vi "Acquire Every Image (178x Smart Camera).vi"() -> ()   [LabVIEW 2023]
doc: "The Acquire Every Image (178x Smart Camera) example performs a high-level grab acquisition and exposes control of the sensor interface for ISC-178x smart cameras. A grab is appropriate for high-speed applications that process only one image at a time.\n\nUse the <B>Sensor Parameters</B> cluster to control attributes related to the sensor. Use the <B>Exposure Time (ms)</B> control to precisely control the amount of time (in milliseconds) that the image sensor is sensitive to light. Use the <B>Gain</B> control to determine the gain of the camera. Use the <B>Reverse X</B> and <B>Reverse Y</B> to flip the image horizontally or vertically.\n\nUse the <B>Lighting Parameters</B> cluster to control the strobe and lighting intensity raw analog output value. The strobe output signal can be output on any ISO output line and is precisely synchronized with the exposure of the image sensor. This guarantees that the light is on for the duration of the image exposure period. The <B>Lighting Intensity Raw</B> is an analog output that can adjust the intensity of a light. \n\nUse the <B>Trigger Parameters</B> cluster to configure the trigger mode of the acquisition. These settings must be configured before running the VI because they are ignored while the acquisition is active."
uses:
  <vilib>/vision/driver/IMAQdx.llb/IMAQdx Buffer Number Mode.ctl
  <vilib>/vision/driver/NI_Vision_Acquisition_Software.lvlib
  <resource>/objmgr/imaqdx.rc
panel:
  in  "SW Trigger":bool
  in  "Trigger Parameters":T1={"Trigger Mode"="Off", "Trigger Source"="Input 0", "Trigger Activation"="Rising Edge", "Acquisition Frame Rate"=1.0, "Timeout (ms)"=5000, "Trigger Delay (us)"=0.0} {"Trigger Delay (us)" min=0.0 max=0.0; "Acquisition Frame Rate" min=0.25 max=293.0}
  in  "Lighting Parameters":T2={"Strobe ISO Output Line"="Off", "Lighting Intensity Raw"=0} {"Lighting Intensity Raw" max=255 step=1 scale=0.0..255.0}
  in  "Color Parameters":T3 {"Blue Gain" scale=0.0..3.99; "Green Gain" scale=0.0..3.99; "Red Gain" scale=0.0..3.99}
  in  "Sensor Parameters":T4={"Exposure Time (ms)"=8.128, "Gain"=0.0, "Reverse X"=FALSE, "Reverse Y"=FALSE} {"Gain" min=0.0 max=255.0; "Exposure Time (ms)" min=0.0 max=4200.0 scale=0.05..4200.0 scale format="%#_1f"}
  in  "Camera Name":refnum<k21> caption="IMAQdx Session"
  out "Image":T5(plugin-control)
  out "Frame Rate":dbl=61.507936507936506 max=294.0
  in  "Stop":bool
  # "Overview: Demonstrates how to perform a high-level grab acquisition and control of the sensor interface for ISC-178x smart camera.  \nRequirements: Vision Acquisition Software, ISC-178x smart camera.\nInstructions: \n1. Open a new LabVIEW Project by selecting Project»Create Project. Select Add this VI when prompted to add this VI to the project.\n2. Right click on the top-level project item in the tree and select New»Targets and Devices\n3. Select the ISC-178x smart camera you want to run this example with, and click OK.\n4. Drag this VI from My Computer to the smart camera target.\n5. Double click on the example under the smart camera, select the Camera Name, and run the VI."
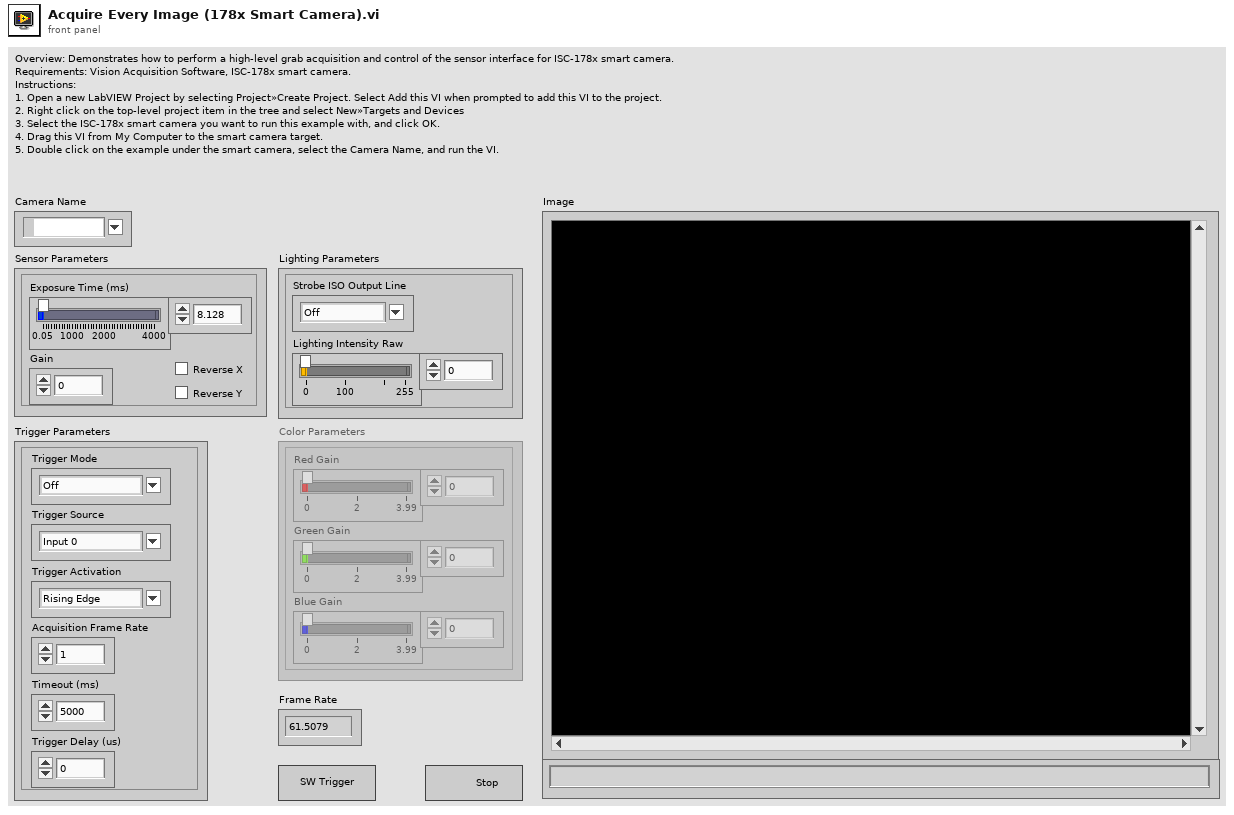
[diagram p1: front panel]
types:
  T1 = cluster{"Trigger Mode":string, "Trigger Source":string, "Trigger Activation":string, "Acquisition Frame Rate":dbl, "Timeout (ms)":u32, "Trigger Delay (us)":dbl}
  T2 = cluster{"Strobe ISO Output Line":string, "Lighting Intensity Raw":u32}
  T3 = cluster{"Red Gain":dbl, "Green Gain":dbl, "Blue Gain":dbl}
  T4 = cluster{"Exposure Time (ms)":dbl, "Gain":dbl, "Reverse X":bool, "Reverse Y":bool}
  T5 = typedef "IMAQ Image.ctl" = refnum<image>
  T6 = enum8{"Enabled", "Disabled", "Disabled and Grayed Out"}
  T7 = typedef "IMAQdx.ctl" = refnum<k21>
  T8 = typedef "NI_Vision_Acquisition_Software.lvlib/IMAQdx Buffer Number Mode.ctl" = enum32{"Next", "Last", "Buffer Number", "Every", "Last New"}
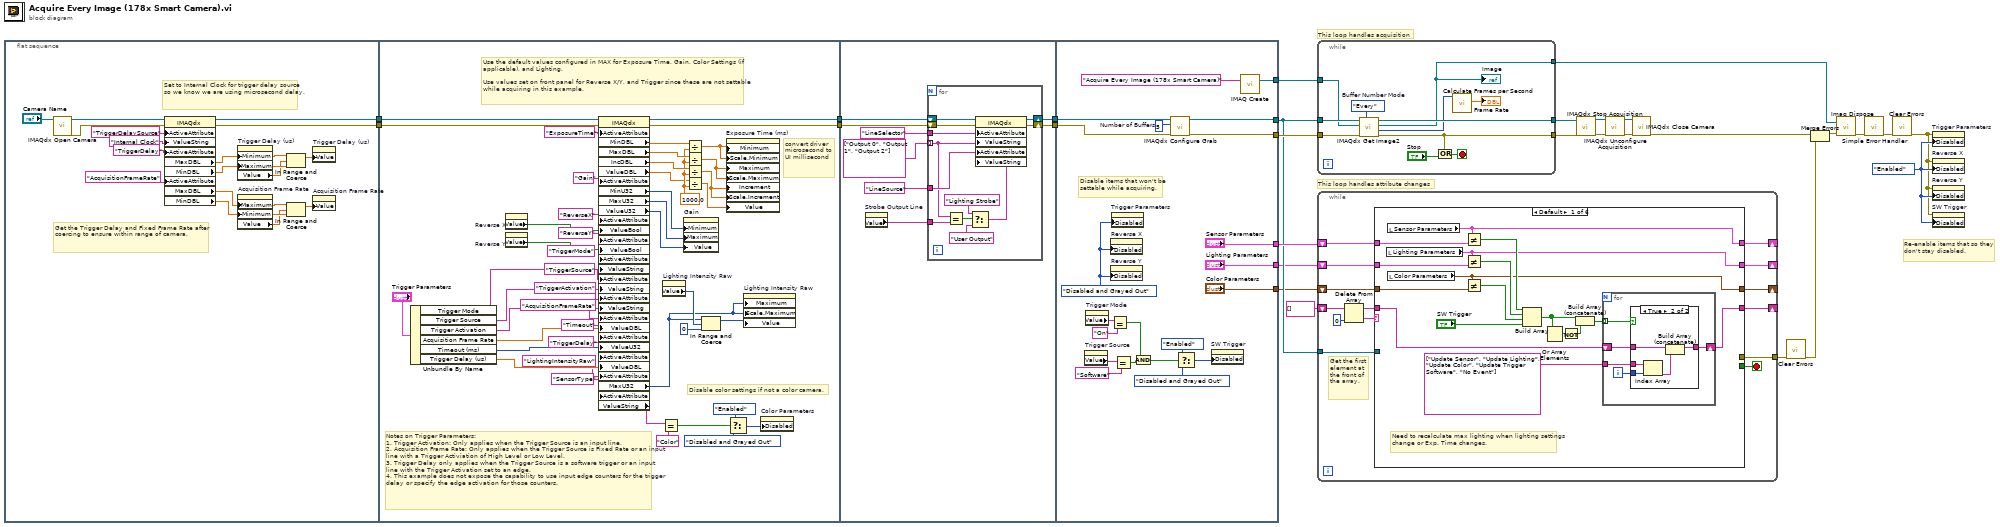
[diagram p0: block diagram]
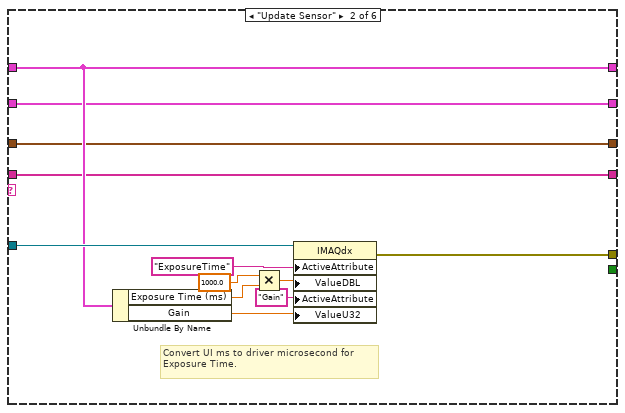
[diagram p3: hidden frame]
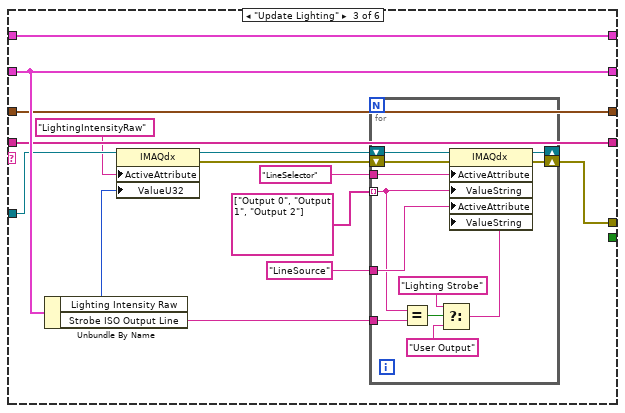
[diagram p4: hidden frame]
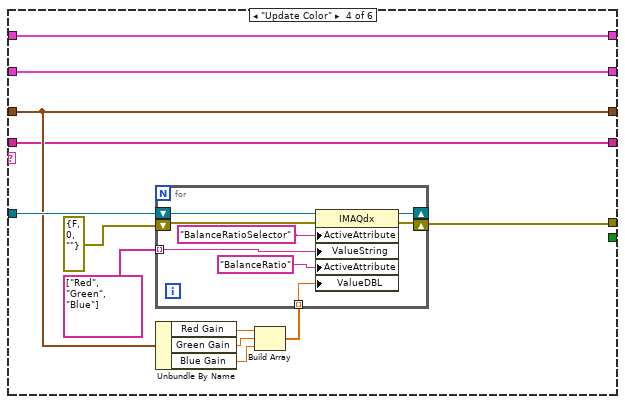
[diagram p5: hidden frame]
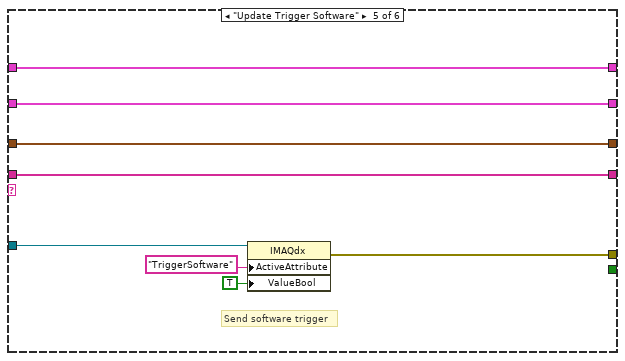
[diagram p6: hidden frame]
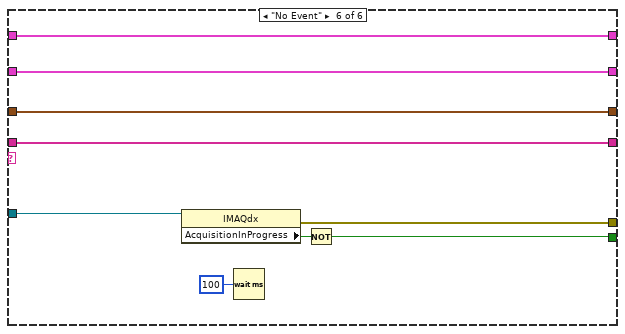
[diagram p7: hidden frame]
diagram:
  w16 = T6."Enabled" ("Disabled")
  # "Re-enable items that so they don't stay disabled."
  # "This loop handles acquisition"
  # "This loop handles attribute changes"
  n1 = flat-sequence {
    tunnel: [w32] -> w23
    tunnel: [w34] -> w22
    tunnel: w23 -> [w63]
    tunnel: [w62] -> w4
    tunnel: w22 -> [w82]
    tunnel: [w76] -> w2
    tunnel: w4 -> [w100]
    tunnel: [w98] -> w3
    tunnel: w2 -> [w99]
    tunnel: [w97] -> w1
    tunnel: w3 -> [w117]
    tunnel: [w116] -> w26
    tunnel: [w115] -> w28
    tunnel: ["Sensor Parameters"] -> w27
    tunnel: ["Lighting Parameters"] -> w25
    tunnel: ["Color Parameters"] -> w24
    tunnel: w1 -> [w114]
    tunnel: [w119] -> w21
    frame #0 {
      # "Get the Trigger Delay and Fixed Frame Rate after coercing to ensure within range of camera."
      # "Set to Internal Clock for trigger delay source so we know we are using microsecond delay."
      n2 = call <vilib>:"IMAQdx Open Camera.vi"("Session In"="Camera Name") -> ("error out"=w29:errorcluster, "Session Out"=w30:T7)  [unwired: 2 in, 7 out]
      n3 = property class="IMAQdx"(reference=w30, error in=w29, "ActiveAttribute"="TriggerDelaySource", "ValueString"="Internal Clock", "ActiveAttribute"="TriggerDelay", "ActiveAttribute"="AcquisitionFrameRate") -> (reference out=w32:T7, error out=w34:errorcluster, "MaxDBL"=w42:dbl, "MinDBL"=w41:dbl, "MaxDBL"=w37:dbl, "MinDBL"=w36:dbl)
      n4 = property on="Trigger Delay (us)" class="DigNum (strict)"("Minimum"=w42, "Maximum"=w41) -> ("Value"=w40:dbl)  [unwired: 2 in, 2 out]
      n5 = property on="Acquisition Frame Rate" class="DigNum (strict)"("Maximum"=w37, "Minimum"=w36) -> ("Value"=w35:dbl)  [unwired: 2 in, 2 out]
      n6 = In Range and Coerce(upper limit=w42, x=w40, lower limit=w41) -> (coerced(x)=w39:dbl)  [unwired: 1 out]
      n7 = In Range and Coerce(upper limit=w37, x=w35, lower limit=w36) -> (coerced(x)=w33:dbl)  [unwired: 1 out]
      n8 = property on="Trigger Delay (us)" class="DigNum (strict)"("Value"=w39) -> ()  [unwired: 2 in, 2 out]
      n9 = property on="Acquisition Frame Rate" class="DigNum (strict)"("Value"=w33) -> ()  [unwired: 2 in, 2 out]
    }
    frame #1 {
      w70 = 1000.0 ("y")
      # "Notes on Trigger Parameters:\n1. Trigger Activation: Only applies when the Trigger Source is an input line.\n2. Acquisition Frame Rate: Only applies when the Trigger Source is Fixed Rate or an input line with a Trigger Activiation of High Level or Low Level. \n3. Trigger Delay only applies when the Trigger Source is a software trigger or an input line with the Trigger Activation set to an edge.\n4. This example does not expose the capability to use input edge counters for the trigger delay or specify the edge activation for those counters."
      # "convert driver microsecond to UI millisecond"
      # "Disable color settings if not a color camera."
      # "Use the default values configured in MAX for Exposure Time, Gain, Color Settings (if applicable), and Lighting.\n\nUse values set on front panel for Reverse X/Y, and Trigger since these are not settable while acquiring in this example."
      n10 = Unbundle By Name("Trigger Parameters") -> ("Trigger Mode"=w56:string, "Trigger Source"=w59:string, "Trigger Activation"=w46:string, "Acquisition Frame Rate"=w49:dbl, "Timeout (ms)"=w58:u32, "Trigger Delay (us)"=w57:dbl)
      n11 = property on="Reverse X" class="Bool (strict)"() -> ("Value"=w86:bool)  [unwired: 2 in, 2 out]
      n12 = property on="Reverse Y" class="Bool (strict)"() -> ("Value"=w85:bool)  [unwired: 2 in, 2 out]
      n13 = property class="IMAQdx"(reference=w63, error in=w82, "ActiveAttribute"="ExposureTime", "ActiveAttribute"="Gain", "ActiveAttribute"="ReverseX", "ValueBool"=w86, "ActiveAttribute"="ReverseY", "ValueBool"=w85, "ActiveAttribute"="TriggerMode", "ValueString"=w56, "ActiveAttribute"="TriggerSource", "ValueString"=w59, "ActiveAttribute"="TriggerActivation", "ValueString"=w46, "ActiveAttribute"="AcquisitionFrameRate", "ValueDBL"=w49, "ActiveAttribute"="Timeout", "ValueU32"=w58, "ActiveAttribute"="TriggerDelay", "ValueDBL"=w57, "ActiveAttribute"="LightingIntensityRaw", "ActiveAttribute"="SensorType") -> (reference out=w62:T7, error out=w76:errorcluster, "MinDBL"=w74:dbl, "MaxDBL"=w73:dbl, "IncDBL"=w72:dbl, "ValueDBL"=w50:dbl, "MinU32"=w91:u32, "MaxU32"=w90:u32, "ValueU32"=w89:u32, "MaxU32"=w51:u32, "ValueString"=w54:string)
      n14 = Equal?(x=w54, y="Color" ("x")) -> (x = y?=w75:bool)
      n15 = property on="Lighting Intensity Raw" class="Slide (strict)"() -> ("Value"=w55:u32)  [unwired: 2 in, 2 out]
      n16 = property on="Gain" class="DigNum (strict)"("Minimum"=w91, "Maximum"=w90, "Value"=w89) -> ()  [unwired: 2 in, 2 out]
      n17 = Divide(x=w74, y=w70) -> (x/y=w69:dbl)
      n18 = Divide(x=w73, y=w70) -> (x/y=w61:dbl)
      n19 = Divide(x=w72, y=w70) -> (x/y=w68:dbl)
      n20 = Divide(x=w50, y=w70) -> (x/y=w67:dbl)
      n21 = In Range and Coerce(upper limit=w51, x=w55, lower limit=u32 0) -> (coerced(x)=w78:u32)  [unwired: 1 out]
      n22 = property on="Exposure Time (ms)" class="Slide (strict)"("Minimum"=w69, "Scale.Minimum"=w69, "Maximum"=w61, "Scale.Maximum"=w61, "Increment"=w68, "Scale.Increment"=w68, "Value"=w67) -> ()  [unwired: 2 in, 2 out]
      n23 = Select(t=T6."Enabled" ("Disabled"), s=w75, f=T6."Disabled and Grayed Out" ("Disabled")) -> (s? t:f=w65:T6)
      n24 = property on="Lighting Intensity Raw" class="Slide (strict)"("Maximum"=w51, "Scale.Maximum"=w51, "Value"=w78) -> ()  [unwired: 2 in, 2 out]
      n25 = property on="Color Parameters" class="Clust (strict)"("Disabled"=w65) -> ()  [unwired: 2 in, 2 out]
    }
    frame #2 {
      n26 = property on="Strobe Output Line" class="CmbBox"() -> ("Value"=w93:string)  [unwired: 2 in, 2 out]
      n27 = for {
        shift-right: [w110] -> w98
        shift-left: w100 -> [w112]
        shift-right: [w109] -> w97
        shift-left: w99 -> [w111]
        tunnel: "LineSelector" -> [w108]
        tunnel: string[] ["Output 0", "Output 1", "Output 2"] -> [w105] mode=indexing
        tunnel: "LineSource" -> [w107]
        tunnel: w93 -> [w106]
        n28 = Equal?(x=w105, y=w106) -> (x = y?=w104:bool)
        n29 = Select(t="Lighting Strobe", s=w104, f="User Output") -> (s? t:f=w101:string)
        n30 = property class="IMAQdx"(reference=w112, error in=w111, "ActiveAttribute"=w108, "ValueString"=w105, "ActiveAttribute"=w107, "ValueString"=w101) -> (reference out=w110:T7, error out=w109:errorcluster)
      }
    }
    frame #3 {
      w118 = T6."Disabled and Grayed Out" ("Disabled")
      w113 = u32 5  # Number of Buffers
      # "Disable items that won't be settable while acquiring."
      n31 = property on="Trigger Source" class="CmbBox"() -> ("Value"=w128:string)  [unwired: 2 in, 2 out]
      n32 = property on="Trigger Mode" class="CmbBox"() -> ("Value"=w130:string)  [unwired: 2 in, 2 out]
      n33 = property on="Reverse X" class="Bool (strict)"("Disabled"=w118) -> ()  [unwired: 2 in, 2 out]
      n34 = property on="Reverse Y" class="Bool (strict)"("Disabled"=w118) -> ()  [unwired: 2 in, 2 out]
      n35 = Equal?(x=w130, y="On") -> (x = y?=w125:bool)
      n36 = property on="Trigger Parameters" class="Clust (strict)"("Disabled"=w118) -> ()  [unwired: 2 in, 2 out]
      n37 = Equal?(x=w128, y="Software") -> (x = y?=w126:bool)
      n38 = And(x=w125, y=w126) -> (x .and. y?=w124:bool)
      n39 = call <vilib>:"IMAQdx Configure Grab.vi"("error in"=w114, "Number of Buffers"=w113, "Session In"=w117) -> ("error out"=w115:errorcluster, "Session Out"=w116:T7)  [unwired: 7 in]
      n40 = Select(t=T6."Enabled" ("Disabled"), s=w124, f=T6."Disabled and Grayed Out" ("Disabled")) -> (s? t:f=w123:T6)
      n41 = property on="SW Trigger" class="Bool"("Disabled"=w123) -> ()  [unwired: 2 in, 2 out]
      n42 = call "IMAQ Create"("Image Name"="Acquire Every Image (178x Smart Camera)") -> ("New Image"=w119:T5)  [unwired: 3 in, 2 out]
    }
  }
  n43 = while {
    tunnel: [w141] -> w20
    tunnel: w28 -> [w142]
    tunnel: w26 -> [w143]
    tunnel: [w137] -> w19
    tunnel: w21 -> [w136]
    tunnel: [w134] -> w18
    stop <- w144 stop-if-true
    w140 = IMAQdx_Buffer_Number_Mode."Every"  # Buffer Number Mode
    n44 = call <vilib>:"IMAQdx Get Image2.vi"("Buffer Number Mode (Next)"=w140, "error in"=w142, "Image In"=w136, "Session In"=w143) -> ("error out"=w137:errorcluster, "Buffer Number Out"=w135:u32, "Image Out"=w134:T5, "Session Out"=w141:T7)  [unwired: 4 in]
    "Image" <- w134
    n45 = Or(x=w137, y="Stop") -> (x .or. y?=w144:bool)
    n46 = call <vilib>:"Calculate Frames per Second.vi"("Buffer Number"=w135) -> ("Processed Frames/s"=→"Frame Rate":dbl)  [unwired: 8 in, 2 out]
  }
  n47 = while {
    shift-right: [w157] -> _
    shift-left: w27 -> [w158]
    shift-right: [w155] -> _
    shift-left: w25 -> [w148]
    shift-right: [w154] -> _
    shift-left: w24 -> [w147]
    tunnel: w26 -> [w156]
    shift-right: [w146] -> _
    shift-left: string[] [] -> [w151]
    tunnel: [w145] -> w11
    stop <- w153 stop-if-true
    # "Get the first element at the front of the array."
    n48 = Delete From Array(array=w151, index=0) -> (deleted portion=w150:string, array with subset deleted=w149:string[])  [unwired: 1 in]
    n49 = case shown="Default" w150 {
      tunnel: w158 -> [w175 w191 w211 w229 w249 w255]
      tunnel: [w165 w191 w211 w229 w249 w255] -> w157
      tunnel: w156 -> [_ w198 w203 w236 w252 w260]
      tunnel: [w164 w190 w212 w228 w248 w256] -> w155
      tunnel: [w163 w189 w210 w235 w247 w257] -> w154
      tunnel: [_ _ _ _ _ w253] -> w153
      tunnel: w147 -> [w173 w189 w210 w235 w247 w257]
      tunnel: w149 -> [w169 w188 w209 w227 w246 w258]
      tunnel: w148 -> [w174 w190 w212 w228 w248 w256]
      tunnel: [w161 w188 w209 w227 w246 w258] -> w146
      tunnel: [_ w187 w205 w225 w245 w254] -> w145
      frame Default {
        # "Need to recalculate max lighting when lighting settings change or Exp. Time changes."
        n50 = local read "Lighting Parameters"() -> (w164:T2)
        n51 = local read "Sensor Parameters"() -> (w165:T4)
        n52 = local read "Color Parameters"() -> (w163:T3)
        n53 = Not Equal?(x=w165, y=w175) -> (x != y?=w168:bool)
        n54 = Not Equal?(x=w164, y=w174) -> (x != y?=w167:bool)
        n55 = Not Equal?(x=w163, y=w173) -> (x != y?=w172:bool)
        n56 = Build Array(w168, w167, w172, "SW Trigger") -> (w171:bool[])
        n57 = Or Array Elements(Boolean array=w171) -> (logical OR=w160:bool)
        n58 = Not(x=w160) -> (.not. x?=w159:bool)
        n59 = Build Array (concatenate)(w171, w159) -> (w170:bool[])
        n60 = for {
          tunnel: w170 -> [w180] mode=indexing
          shift-right: [w178] -> w161
          shift-left: w169 -> [w179]
          tunnel: string[] ["Update Sensor", "Update Lighting", "Update Color", "Update Trigger Software", "No Event"] -> [w177]
          i -> [w176]
          n61 = case shown="True" w180 {
            tunnel: w179 -> [w181 w186]
            tunnel: w176 -> [_ w185]
            tunnel: [w181 w183] -> w178
            tunnel: w177 -> [_ w182]
            frame False {
            }
            frame True {
              n62 = Index Array(array=w182, index=w185) -> (element=w184:string)
              n63 = Build Array (concatenate)(w186, w184) -> (w183:string[])
            }
          }
        }
      }
      frame "Update Sensor" {
        # "Convert UI ms to driver microsecond for Exposure Time."
        n64 = Unbundle By Name(w191) -> ("Exposure Time (ms)"=w193:dbl, "Gain"=w197:dbl)
        n65 = Multiply(x=1000.0, y=w193) -> (x*y=w194:dbl)
        n66 = property class="IMAQdx"(reference=w198, "ActiveAttribute"="ExposureTime", "ValueDBL"=w194, "ActiveAttribute"="Gain", "ValueU32"=w197) -> (error out=w187:errorcluster)  [unwired: 1 in, 1 out]
      }
      frame "Update Lighting" {
        n67 = Unbundle By Name(w212) -> ("Lighting Intensity Raw"=w199:u32, "Strobe ISO Output Line"=w204:string)
        n68 = property class="IMAQdx"(reference=w203, "ActiveAttribute"="LightingIntensityRaw", "ValueU32"=w199) -> (reference out=w202:T7, error out=w201:errorcluster)  [unwired: 1 in]
        n69 = for {
          shift-right: [w222] -> _
          shift-left: w202 -> [w224]
          shift-right: [w221] -> w205
          shift-left: w201 -> [w223]
          tunnel: "LineSelector" -> [w220]
          tunnel: string[] ["Output 0", "Output 1", "Output 2"] -> [w217] mode=indexing
          tunnel: "LineSource" -> [w219]
          tunnel: w204 -> [w218]
          n70 = Equal?(x=w217, y=w218) -> (x = y?=w216:bool)
          n71 = Select(t="Lighting Strobe", s=w216, f="User Output") -> (s? t:f=w213:string)
          n72 = property class="IMAQdx"(reference=w224, error in=w223, "ActiveAttribute"=w220, "ValueString"=w217, "ActiveAttribute"=w219, "ValueString"=w213) -> (reference out=w222:T7, error out=w221:errorcluster)
        }
      }
      frame "Update Color" {
        n73 = Unbundle By Name(w235) -> ("Red Gain"=w233:dbl, "Green Gain"=w232:dbl, "Blue Gain"=w231:dbl)
        n74 = Build Array(w233, w232, w231) -> (w230:dbl[])
        n75 = for {
          tunnel: string[] ["Red", "Green", "Blue"] -> [w241] mode=indexing
          tunnel: w230 -> [w240] mode=indexing
          shift-right: [w239] -> _
          shift-left: w236 -> [w244]
          shift-right: [w237] -> w225
          shift-left: errorcluster {"status"=FALSE, "code"=0, "source"=""} ("error out") -> [w238]
          n76 = property class="IMAQdx"(reference=w244, error in=w238, "ActiveAttribute"="BalanceRatioSelector", "ValueString"=w241, "ActiveAttribute"="BalanceRatio", "ValueDBL"=w240) -> (reference out=w239:T7, error out=w237:errorcluster)
        }
      }
      frame "Update Trigger Software" {
        # "Send software trigger"
        n77 = property class="IMAQdx"(reference=w252, "ActiveAttribute"="TriggerSoftware", "ValueBool"=TRUE) -> (error out=w245:errorcluster)  [unwired: 1 in, 1 out]
      }
      frame "No Event" {
        n78 = property class="IMAQdx"(reference=w260) -> (error out=w254:errorcluster, "AcquisitionInProgress"=w259:bool)  [unwired: 1 in, 1 out]
        n79 = Wait (ms)(milliseconds to wait=u32 100) -> ()  [unwired: 1 out]
        n80 = Not(x=w259) -> (.not. x?=w253:bool)
      }
    }
  }
  n81 = call <vilib>:"IMAQdx Stop Acquisition.vi"("error in"=w19, "Session In"=w20) -> ("error out"=w15:errorcluster, "Session Out"=w14:T7)  [unwired: 8 out]
  n82 = call <vilib>:"IMAQdx Unconfigure Acquisition.vi"("error in"=w15, "Session In"=w14) -> ("error out"=w12:errorcluster, "Session Out"=w13:T7)  [unwired: 8 out]
  n83 = call <vilib>:"IMAQdx Close Camera.vi"("error in"=w12, "Session In"=w13) -> ("error out"=w10:errorcluster)  [unwired: 9 out]
  n84 = call <vilib>:"Clear Errors.vi"("error in (no error)"=w11) -> ("error out"=w9:errorcluster)  [unwired: 5 in, 1 out]
  n85 = Merge Errors(w10, w9) -> (w8:errorcluster)
  n86 = call "Imaq Dispose"("Image"=w18, "error in (no error)"=w8) -> ("error out"=w6:errorcluster)  [unwired: 4 in]
  n87 = call <vilib>:"Simple Error Handler.vi"("error in (no error)"=w6) -> ("error out"=w5:errorcluster)  [unwired: 4 in, 4 out]
  n88 = call <vilib>:"Clear Errors.vi"("error in (no error)"=w5) -> ("error out"=w7:errorcluster)  [unwired: 5 in, 1 out]
  n89 = property on="Trigger Parameters" class="Clust (strict)"(error in=w7, "Disabled"=w16) -> ()  [unwired: 1 in, 2 out]
  n90 = property on="Reverse X" class="Bool (strict)"(error in=w7, "Disabled"=w16) -> ()  [unwired: 1 in, 2 out]
  n91 = property on="Reverse Y" class="Bool (strict)"(error in=w7, "Disabled"=w16) -> ()  [unwired: 1 in, 2 out]
  n92 = property on="SW Trigger" class="Bool"(error in=w7, "Disabled"=w16) -> ()  [unwired: 1 in, 2 out]
